vi "BuildTimeArray.vi"(1 "Time Increment (dt)":dbl, 2 "Data Array (y-values)":dbl[](array[numeric]), 3 "Start Time (t_o)":dbl) -> (0 "Time Array (x-values)":dbl[](array[numeric]))   [LabVIEW 2011]
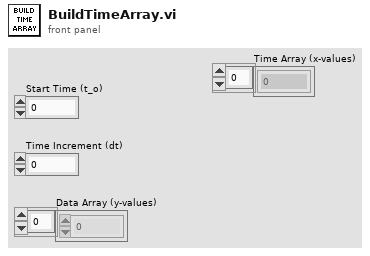
[diagram p1: front panel]
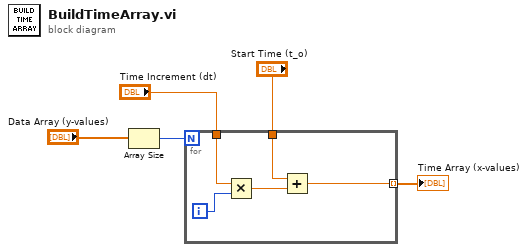
[diagram p0: block diagram]
diagram:
  n1 = Array Size(array="Data Array (y-values)") -> (size(s)=w2:i32)
  n2 = for {
    N: w2 -> [_]
    tunnel: "Time Increment (dt)" -> [w9]
    tunnel: "Start Time (t_o)" -> [w8]
    tunnel: [w6] -> w1 mode=indexing
    i -> [w10]
    n3 = Multiply(x=w9, y=w10) -> (x*y=w7:dbl)
    n4 = Add(x=w8, y=w7) -> (x+y=w6:dbl)
  }
  "Time Array (x-values)" <- w1
